vi "E2 Lookup Table Initialize.vi"(8 "error in (no error)":errorcluster, 11 "Lookup Table File":path=path "C:/Users/schalla/Desktop/LUT/LUT.csv") -> (2 "Array of XY Data Points":cluster{"X":dbl, "Y":dbl}[](array[cluster]))   [LabVIEW 2015]
uses:
  <vilib>/Utility/file.llb/Read From Spreadsheet File (string).vi
panel:
  # "INPUTS"
  # "OUTPUTS"
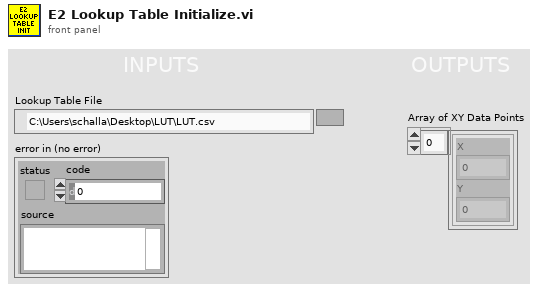
[diagram p1: front panel]
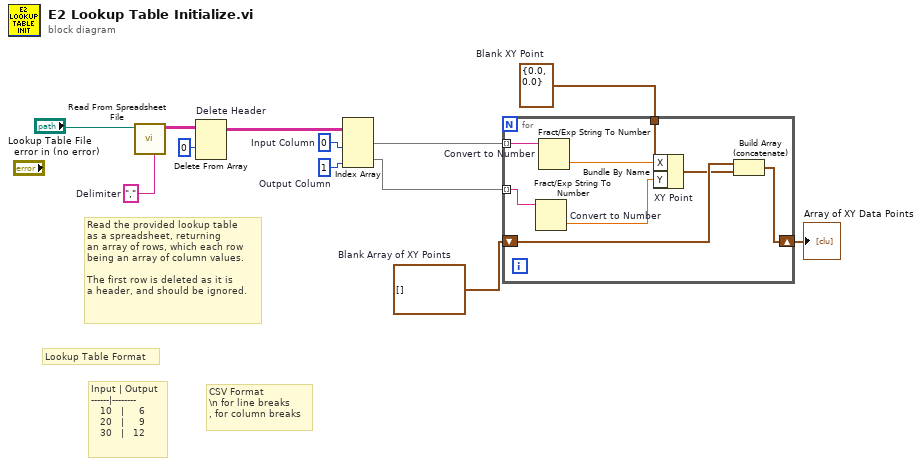
[diagram p0: block diagram]
diagram:
  w2 = cluster{"X":dbl, "Y":dbl} {"X"=0.0, "Y"=0.0}  # Blank XY Point
  w3 = cluster{"X":dbl, "Y":dbl}[] []  # Blank Array of XY Points
  w6 = 1  # Output Column
  w7 = 0  # Input Column
  w12 = ","  # Delimiter
  # "CSV Format\n\\n for line breaks\n, for column breaks"
  # "Input | Output\n------|--------\n   10   |     6\n   20   |     9\n   30   |   12"
  # "Lookup Table Format"
  # "Read the provided lookup table\nas a spreadsheet, returning\nan array of rows, which each row\nbeing an array of column values.\n\nThe first row is deleted as it is\na header, and should be ignored."
  n1 = call-poly <vilib>:"Read From Spreadsheet File.vi"("delimiter (\\t)"=w12, "file path (dialog if empty)"="Lookup Table File") -> ("all rows"=w11:string[][])  [unwired: 5 in, 4 out]
  n2 = Delete From Array "Delete Header"(array=w11, index (row)=0) -> (array with subset deleted=w8:string[][])  [unwired: 2 in, 1 out]
  n3 = Index Array(array=w8, index (col) #1=w7, index (col) #2=w6) -> (element #1=w5:string[], element #2=w4:string[])  [unwired: 2 in]
  n4 = for {
    tunnel: w5 -> [w20] mode=indexing
    tunnel: w4 -> [w19] mode=indexing
    shift-right: [w13] -> w1
    shift-left: w3 -> [w18]
    tunnel: w2 -> [w17]
    n5 = Fract/Exp String To Number "Convert to Number"(string=w19) -> (number=w15:dbl)  [unwired: 3 in, 1 out]
    n6 = Fract/Exp String To Number "Convert to Number"(string=w20) -> (number=w16:dbl)  [unwired: 3 in, 1 out]
    n7 = Bundle By Name "XY Point"(cluster=w17, "X"=w16, "Y"=w15) -> (w14:cluster{"X":dbl, "Y":dbl})
    n8 = Build Array (concatenate)(w18, w14) -> (w13:cluster{"X":dbl, "Y":dbl}[])
  }
  "Array of XY Data Points" <- w1
